vi "_009.vi"() -> ()   [LabVIEW 2024]
panel:
  out "deleted portion":dbl[](array[numeric])
  out "array w/ subset deleted":dbl[](array[numeric])
  in  "length":i32
  in  "index":i32
  in  "array":dbl[](array[numeric])
  out "output array":dbl[](array[numeric])
  in  "new element/subarray":dbl
  in  "index":i32
  in  "array":dbl[](array[numeric])
  out "output array":dbl[](array[numeric])
  in  "new element/subarray":dbl
  in  "index":i32
  in  "array":dbl[](array[numeric])
  in  "index":i32
  out "element":dbl
  in  "array":dbl[](array[numeric])
  out "size(s)":i32
  in  "array":dbl[](array[numeric])
  # "ARRAY"
  # "Array Size :"
  # "Index Array :"
  # "Replace Array Subset :"
  # "Insert into Array :"
  # "Delete From Array :"
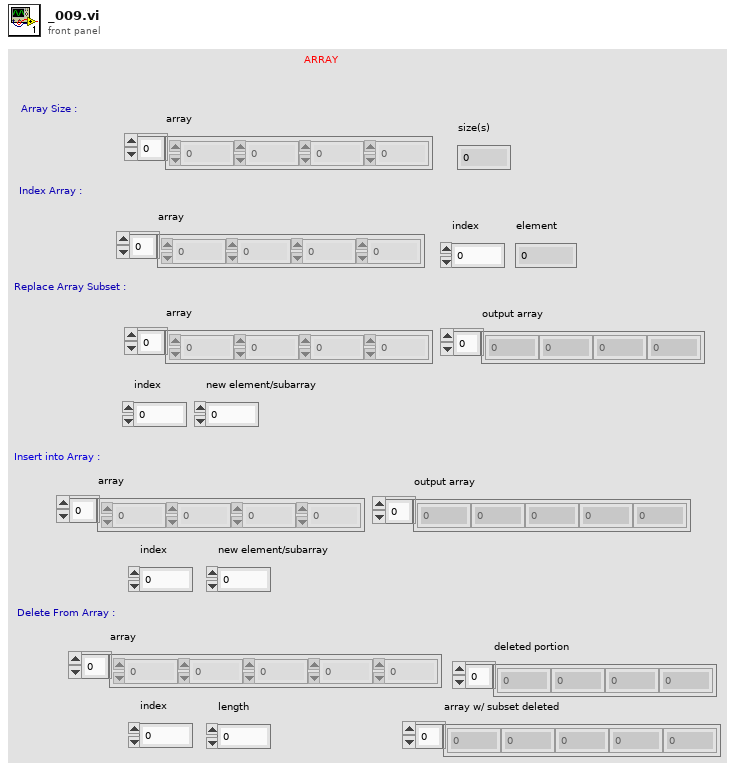
[diagram p1: front panel]
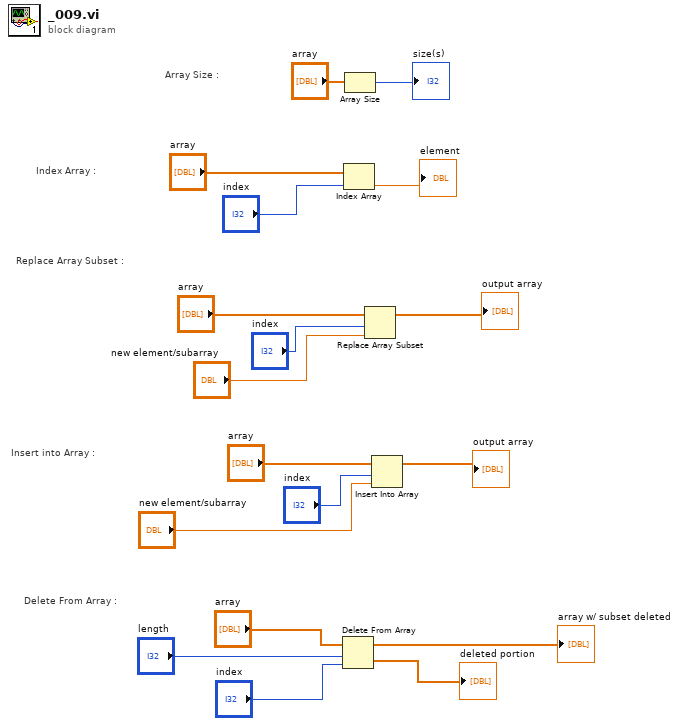
[diagram p0: block diagram]
diagram:
  # "Delete From Array :"
  # "Insert into Array :"
  # "Replace Array Subset :"
  # "Index Array :"
  # "Array Size :"
  n1 = Delete From Array "Delete From Array"(array="array", length="length", index="index") -> (deleted portion=→"deleted portion":dbl[], array with subset deleted=→"array w/ subset deleted":dbl[])
  n2 = Index Array "Index Array"(array="array", index="index") -> (element=→"element":dbl)
  n3 = Array Size(array="array") -> (size(s)=→"size(s)":i32)
  n4 = Replace Array Subset "Replace Array Subset"(array="array", new element="new element/subarray", index="index") -> (→"output array":dbl[])
  n5 = Insert Into Array "Insert Into Array"(array="array", index="index", new element="new element/subarray") -> (→"output array":dbl[])
